vi "VSI Write Read Bits.vi"(5 "ReadBitsNum":i32, 6 "pReadBitStr":string, 7 "pWriteBitStr":string, 9 "SPIIndex":i32, 10 "DevIndex":i32, 11 "DevType":i32) -> (2 "function return":i32, 3 "pWriteBitStr out":string, 4 "pReadBitStr out":string)   [LabVIEW 2010, in "ControlSPI.lvlib"]
doc: "int WINAPI VSI_WriteReadBits(int DevType,int DevIndex,int SPIIndex,unsigned char *pWriteBitStr,unsigned char *pReadBitStr,int ReadBitsNum);"
uses:
  ControlSPI.lvlib
  ControlSPI/Ginkgo_Driver.dll
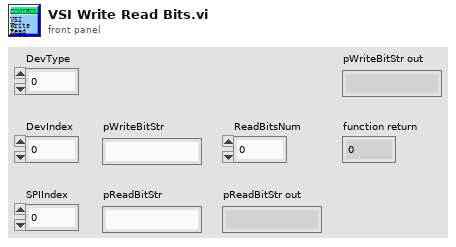
[diagram p1: front panel]
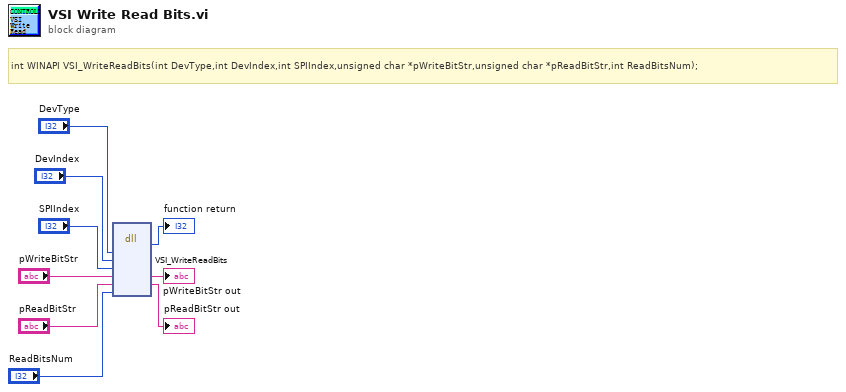
[diagram p0: block diagram]
diagram:
  # "int WINAPI VSI_WriteReadBits(int DevType,int DevIndex,int SPIIndex,unsigned char *pWriteBitStr,unsigned char *pReadBitStr,int ReadBitsNum);"
  n1 = dll-call lib="E:/Project/vt_ginkgo/truck/Ginkgo Driver/vs2010/Ginkgo_USB-I2C&SPI&CAN_API_v2.0.3.3/lib/labview_32bit/ControlSPI/Ginkgo_Driver.*" fn="VSI_WriteReadBits"("DevType"="DevType", "DevIndex"="DevIndex", "SPIIndex"="SPIIndex", "pWriteBitStr"="pWriteBitStr", "pReadBitStr"="pReadBitStr", "ReadBitsNum"="ReadBitsNum") -> (→"function return":i32, "pWriteBitStr"=→"pWriteBitStr out":string, "pReadBitStr"=→"pReadBitStr out":string)  [unwired: 7 in, 2 out]
